vi "CheckDSNConnection.vi"(3 "ConnectionString":string="DSN=trestanques;") -> (0 "error out":errorcluster)   [LabVIEW 2010]
doc: "This example opens a connection to a database specified by the Connection string (replace the DNS name with your database) inserts a new row into the table \"myOtherTable\" (replace the SQL string with your own SQL query)."
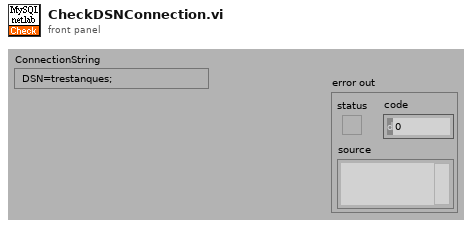
[diagram p1: front panel]
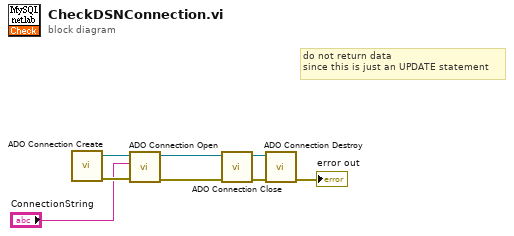
[diagram p0: block diagram]
diagram:
  # "do not return data\nsince this is just an UPDATE statement"
  n1 = call "ADO Connection Create.vi"() -> ("error out"=w7:errorcluster, "ADODB._Connection Out"=w8:refnum<k7>)  [unwired: 1 in, 9 out]
  n2 = call "ADO Connection Open.vi"("error in (no error)"=w7, "ConnectionString"="ConnectionString", "ADODB._Connection In"=w8) -> ("error out"=w1:errorcluster, "ADODB._Connection Out"=w2:refnum<k7>)  [unwired: 7 out]
  n3 = call "ADO Connection Close.vi"("error in (no error)"=w1, "ADODB._Connection In"=w2) -> ("error out"=w5:errorcluster, "ADODB._Connection Out"=w4:refnum<k7>)  [unwired: 8 out]
  n4 = call "ADO Connection Destroy.vi"("error in (no error)"=w5, "ADODB._Connection In"=w4) -> ("error out"=→"error out":errorcluster)  [unwired: 9 out]
